vi "Corr CSV Editor.vi"(8 "error in":errorcluster, 11 "File path":path) -> (0 "error out":errorcluster, 3 "path out":path)   [LabVIEW 2013]
doc: "CSV editor."
panel:
  in  "btn save":bool
  in  "btn exit":bool
  in  "Table data":string[][](table)
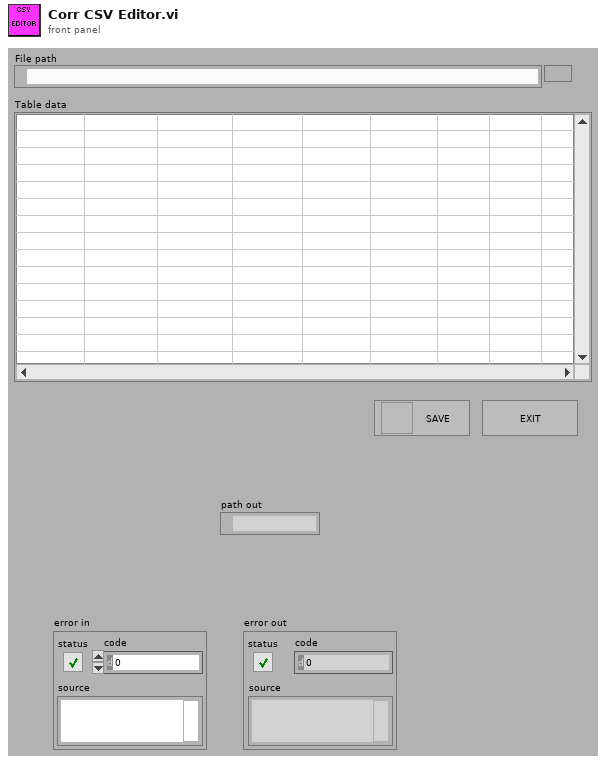
[diagram p1: front panel]
types:
  T1 = typedef "eventvkey.ctl" = enum16{"ASCII", "Enter", "Return", "Shift", "Ctrl", "Alt", "Cmd", "Opt", "Caps", "NumLock", "Clear", "Break", "Up", "Down", "Left", "Right", "Insert", "Delete", "Home", "End", "PageUp", "PageDown", "Escape", "Help", "Pause", "ScrollLock", "F1", "F2", "F3", "F4", "F5", "F6", "F7", "F8", "F9", "F10", "F11", "F12", "F13", "F14", "F15", "F16", "F17", "F18", "F19", "F20", "F21", "F22", "F23", "F24", "Play", "VolumeUp", "VolumeDown", "Mute", "Two Byte Char"}
  T2 = typedef "LVRowAndColumnTypeDef.ctl" = cluster{"Row":i32, "Column":i32}
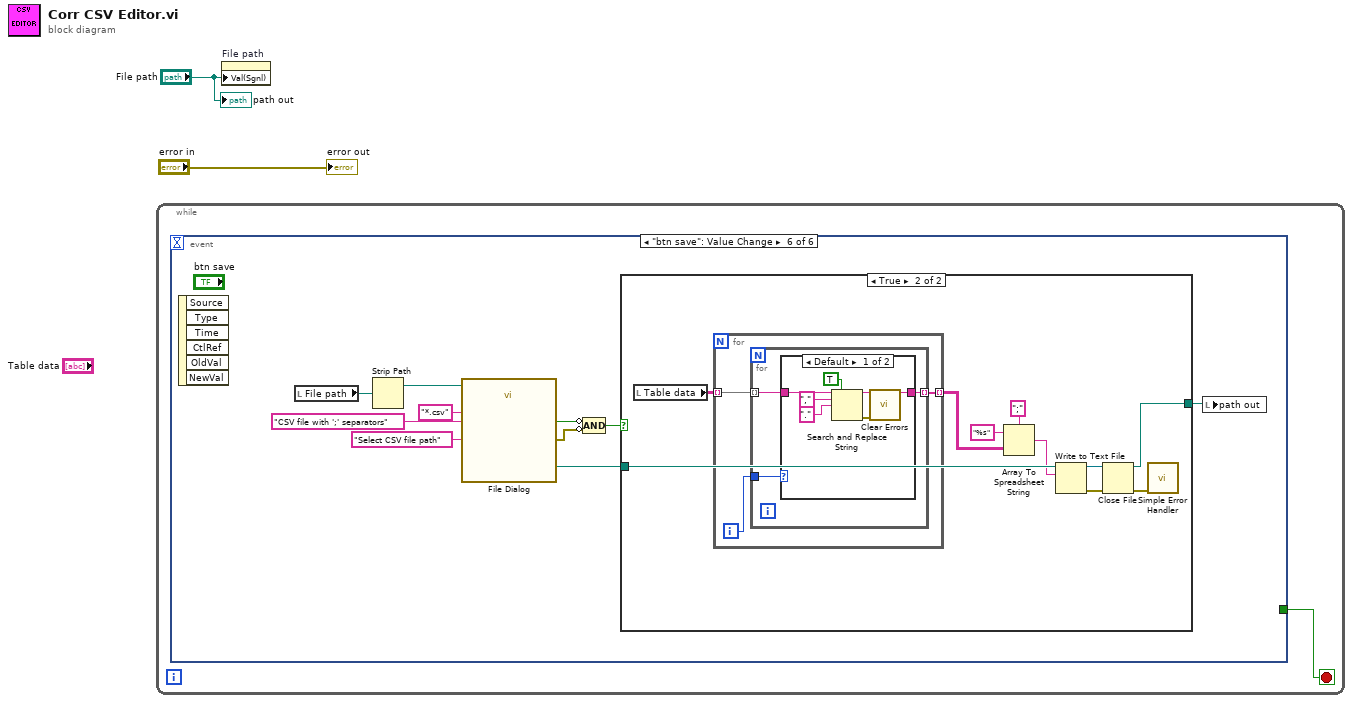
[diagram p0: block diagram]
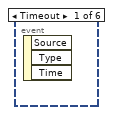
[diagram p2: hidden frame]
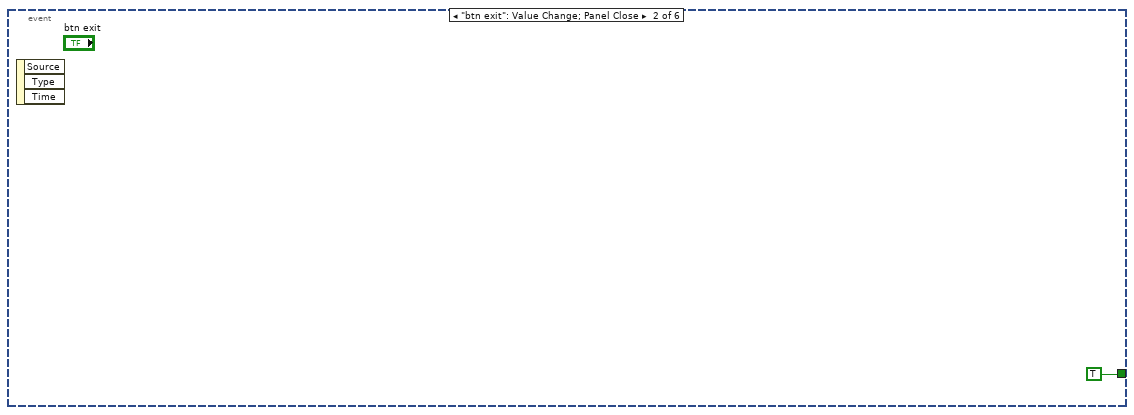
[diagram p3: hidden frame]
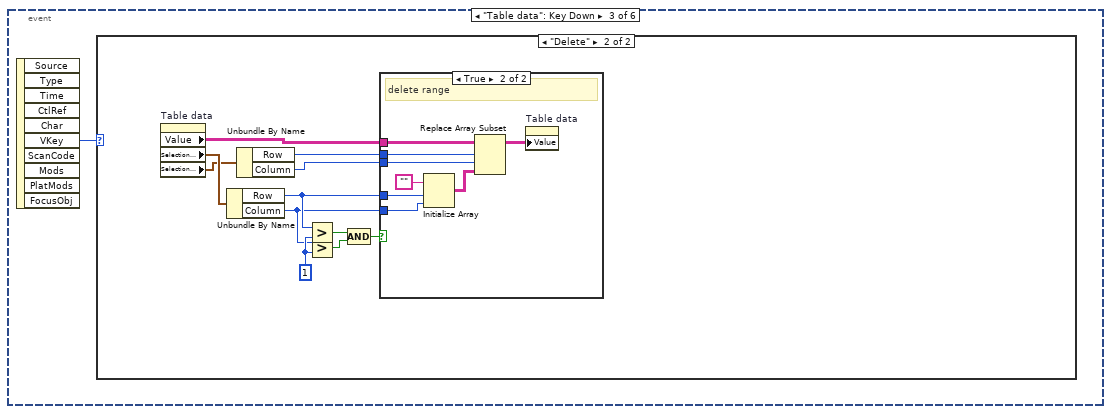
[diagram p4: hidden frame]
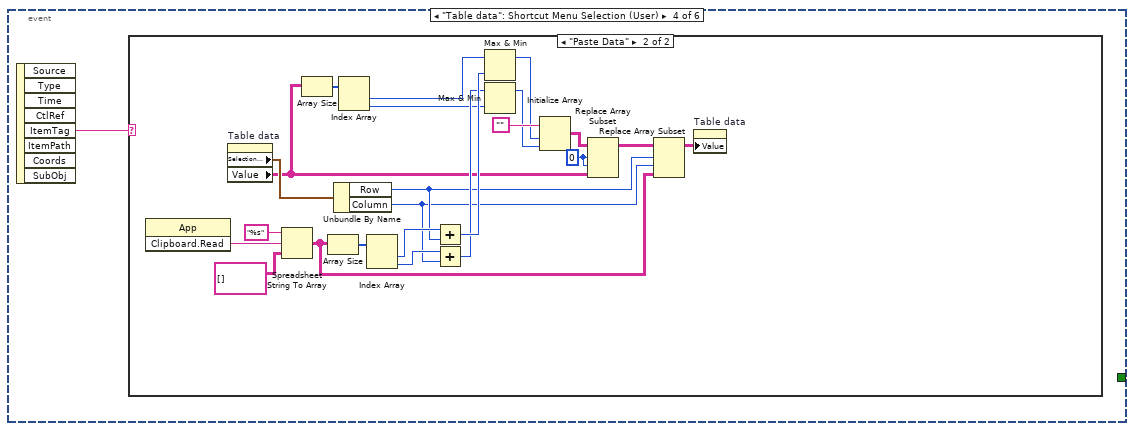
[diagram p7: hidden frame]
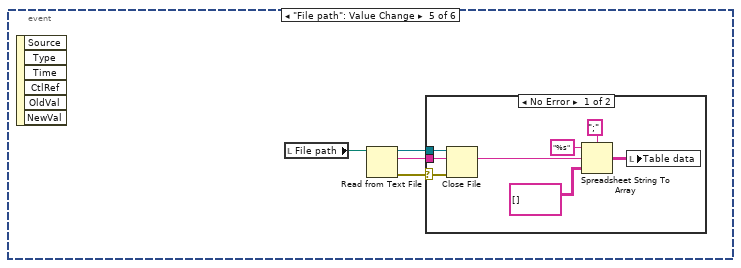
[diagram p9: hidden frame]
diagram:
  n1 = while {
    stop <- w3 stop-if-true
    n2 = event shown="[5] \"btn save\": Value Change" {
      selector: _ -> [_ _ _ _ _ _]
      dyn-events: _ -> [_ _ _ _ _ _]
      timeout: _ -> [_ _ _ _ _ _]
      tunnel: [_ TRUE _ _ _ _] -> w3
      event Timeout {
        n3 = event-data() -> ()  [unwired: 1 in, 3 out]
      }
      event "btn exit": Value Change; Panel Close {
        n4 = event-data() -> ()  [unwired: 1 in, 3 out]
      }
      event "Table data": Key Down {
        n5 = event-data() -> ("VKey"=w5:T1)  [unwired: 1 in, 9 out]
        n6 = case shown="\"Delete\"" w5 {
          frame "ASCII", Default {
          }
          frame "Delete" {
            w15 = 1 ("y")
            n7 = property on="Table data" class="Tbl (strict)"() -> ("Value"=w11:string[][], "Selection Size"=w16:T2, "Selection Start"=w8:T2)  [unwired: 2 in, 2 out]
            n8 = Unbundle By Name(w16) -> ("Row"=w10:i32, "Column"=w9:i32)
            n9 = Unbundle By Name(w8) -> ("Row"=w7:i32, "Column"=w6:i32)
            n10 = Greater?(x=w10, y=w15) -> (0:w14:bool)
            n11 = Greater?(x=w9, y=w15) -> (0:w13:bool)
            n12 = Compound Arithmetic op=AND(w14, w13) -> (w12:bool)
            n13 = case shown="True" w12 {
              tunnel: w11 -> [_ w21]
              tunnel: w10 -> [_ w23]
              tunnel: w9 -> [_ w22]
              tunnel: w7 -> [_ w20]
              tunnel: w6 -> [_ w19]
              frame False {
              }
              frame True {
                # "delete range"
                n14 = Initialize Array("", w23, w22) -> (w18:string[][])
                n15 = Replace Array Subset(array=w21, new element=w18, index (row)=w20, index (col)=w19) -> (w17:string[][])
                n16 = property on="Table data" class="Tbl (strict)"("Value"=w17) -> ()  [unwired: 2 in, 2 out]
              }
            }
          }
        }
      }
      event "Table data": Shortcut Menu Selection (User) {
        n17 = event-data() -> ("ItemTag"=w25:string)  [unwired: 1 in, 7 out]
        n18 = case shown="\"Paste Data\"" w25 {
          frame "False", Default {
          }
          frame "Paste Data" {
            w26 = 0 ("index (row)")
            n19 = invoke class="App" method="Clipboard.Read"() -> ("Read Clipbrd"=w48:string)  [unwired: 3 in, 2 out]
            n20 = property on="Table data" class="Tbl (strict)"() -> ("Selection Start"=w45:T2, "Value"=w32:string[][])  [unwired: 2 in, 2 out]
            n21 = Spreadsheet String To Array(format string="%s", spreadsheet string=w48, array type (2D Dbl)=string[][] []) -> (array=w28:string[][])  [unwired: 1 in]
            n22 = Array Size(array=w32) -> (size(s)=w44:i32[])
            n23 = Array Size(array=w28) -> (size(s)=w42:i32[])
            n24 = Unbundle By Name(w45) -> ("Row"=w30:i32, "Column"=w29:i32)
            n25 = Index Array(array=w44) -> (element #1=w34:i32, element #2=w33:i32)  [unwired: 2 in]
            n26 = Index Array(array=w42) -> (element #1=w41:i32, element #2=w40:i32)  [unwired: 2 in]
            n27 = Add(x=w41, y=w30) -> (x+y=w39:i32)
            n28 = Add(x=w40, y=w29) -> (x+y=w38:i32)
            n29 = Max & Min(x=w34, y=w39) -> (max(x,y)=w37:i32)  [unwired: 1 out]
            n30 = Max & Min(x=w38, y=w33) -> (max(x,y)=w36:i32)  [unwired: 1 out]
            n31 = Initialize Array("", w37, w36) -> (w35:string[][])
            n32 = Replace Array Subset(array=w35, new element=w32, index (row)=w26, index (col)=w26) -> (w31:string[][])
            n33 = Replace Array Subset(array=w31, new element=w28, index (row)=w30, index (col)=w29) -> (w27:string[][])
            n34 = property on="Table data" class="Tbl (strict)"("Value"=w27) -> ()  [unwired: 2 in, 2 out]
          }
        }
      }
      event "File path": Value Change {
        n35 = event-data() -> ()  [unwired: 1 in, 6 out]
        n36 = local read "File path"() -> (w52:path)
        n37 = Read from Text File(file (use dialog)=w52) -> (refnum out=w49:refnum<file>, text=w50:string, error out=w51:errorcluster)  [unwired: 3 in, 1 out]
        n38 = case shown="No Error" w51 {
          selector: w51 -> [w54 _]
          tunnel: w50 -> [w59 _]
          tunnel: w49 -> [w53 _]
          frame No Error {
            n39 = Close File(refnum=w53, error in=w54) -> ()  [unwired: 2 out]
            n40 = Spreadsheet String To Array(delimiter (Tab)=";", format string="%s", spreadsheet string=w59, array type (2D Dbl)=string[][] []) -> (array=w55:string[][])
            n41 = local write "Table data"(w55) -> ()
          }
          frame Error {
          }
        }
      }
      event "btn save": Value Change {
        n42 = event-data() -> ()  [unwired: 1 in, 6 out]
        n43 = local read "File path"() -> (w68:path)
        n44 = Strip Path(path=w68) -> (stripped path=w69:path)  [unwired: 1 out]
        n45 = call "File Dialog"("start path"=w69, "prompt"="Select CSV file path", "pattern (all files)"="*.csv", "pattern label"="CSV file with ';' separators") -> ("selected path"=w61:path, "cancelled"=w64:bool, "error out"=w63:errorcluster)  [unwired: 8 in, 1 out]
        n46 = Compound Arithmetic op=AND(invert w64, invert w63) -> (w62:bool)
        n47 = case shown="True" w62 {
          tunnel: w61 -> [_ w77]
          tunnel: [_ w72] -> w60
          frame False {
          }
          frame True {
            n48 = local read "Table data"() -> (w71:string[][])
            n49 = for {
              tunnel: w71 -> [w82] mode=indexing
              tunnel: [w80] -> w70 mode=indexing
              i -> [w81]
              n50 = for {
                tunnel: w82 -> [w84] mode=indexing
                tunnel: w81 -> [w85]
                tunnel: [w83] -> w80 mode=indexing
                n51 = case shown="Default" w85 {
                  tunnel: [w90 w92] -> w83
                  tunnel: w84 -> [w91 w92]
                  frame Default {
                    n52 = Search and Replace String(replace all?=TRUE ("replace all? (F)"), input string=w91, search string=",", replace string="." ("replace string (\"\")")) -> (result string=w90:string, error out=w86:errorcluster)  [unwired: 4 in, 2 out]
                    n53 = call <vilib>:"Clear Errors.vi"("error in (no error)"=w86) -> ()  [unwired: 6 in, 1 out]
                  }
                  frame 0 {
                  }
                }
              }
            }
            n54 = Array To Spreadsheet String(delimiter (Tab)=";", array=w70, 3:"%s" ("format string")) -> (spreadsheet string=w76:string)
            n55 = Write to Text File(file (use dialog)=w77, text=w76) -> (refnum out=w74:refnum<file>, error out=w75:errorcluster)  [unwired: 2 in, 1 out]
            n56 = Close File(refnum=w74, error in=w75) -> (path=w72:path, error out=w73:errorcluster)
            n57 = call <vilib>:"Simple Error Handler.vi"("error in (no error)"=w73) -> ()  [unwired: 4 in, 5 out]
          }
        }
        n58 = local write "path out"(w60) -> ()
      }
    }
  }
  n59 = property on="File path" class="Path"("Val(Sgnl)"="File path") -> ()  [unwired: 2 in, 2 out]
  "error out" <- "error in"
  "path out" <- "File path"
